vi "logical-operations.vi"() -> ()   [LabVIEW 2020]
panel:
  out "(hi.lo)":u16
  out "x .and. y?":i16
  in  "lo":u16=248
  in  "hi":u16=3
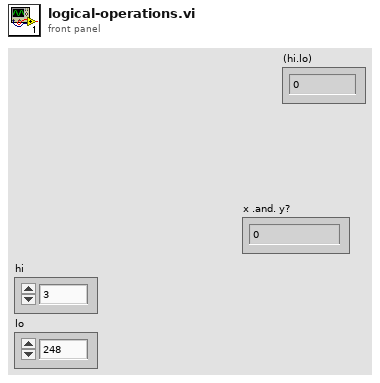
[diagram p1: front panel]
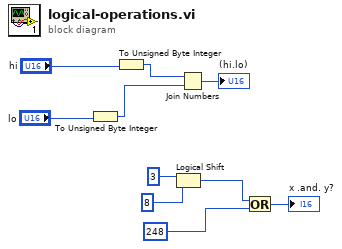
[diagram p0: block diagram]
diagram:
  n1 = To Unsigned Byte Integer(number="lo") -> (unsigned 8bit integer=w2:u8)
  n2 = To Unsigned Byte Integer(number="hi") -> (unsigned 8bit integer=w4:u8)
  n3 = Logical Shift(y=i16 3, x=i16 8) -> (x << y=w8:i16)
  n4 = Join Numbers(hi=w4, lo=w2) -> ((hi.lo)=→"(hi.lo)":u16)
  n5 = Or(x=w8, y=i16 248) -> (x .or. y?=→"x .and. y?":i16)
